vi "PH_4_Pos_Selector.ProcCases.vi"(0 "i ref in":refnum<vi>, 1 "selector":string, 2 "data":i8[](array[numeric]), 3 "call cluster":T1={"Object"="", "Selector"="", "CallType"=enum."synchronous", "Async Object"="", "Async Selector"="", "Data Descriptor"="", "Data"=[], "Error #"=0, "Expire"=0}, 5 "error in":errorcluster) -> (14 "i ref out":refnum<vi>, 17 "answer cluster":T1={"Object"="", "Selector"="", "CallType"=enum."synchronous", "Async Object"="", "Async Selector"="", "Data Descriptor"="", "Data"=[], "Error #"=0, "Expire"=0}, 19 "error out":errorcluster)   [LabVIEW 2014, in "PH_4_Pos_Selector.lvlib"]
doc: "This method is called by a process from within the default case in the event loop. The methods of a class that are linked to events will be called from THIS method. Add your code here."
uses:
  PH_4_Pos_Selector.lvlib
  CSCore/CSSystem/CoreDefs/CoreDefs.call_type.ctl
  CSCore/BaseProcess/BaseProcess.descriptor string definition.ctl
  CSCore/CSSystem/CoreDefs/CoreDefs.rawDataType.ctl
  PH_4_Pos_Selector.Position Selector.ctl
  CSCore/CSSystem/CoreLib/CoreLib.string 2 byte array.vi
  CSCore/CSSystem/CoreLib/CoreLib.byte array 2 short.vi
  PH_AxisGUI_6P/PH_AxisGUI_6P.lvlib
  CSCore/CSSystem/CoreLib/CoreLib.lvlib
  CSCore/BaseProcess/BaseProcess.lvlib
  CSCore/CAEObj/CAEObj.lvlib
  PH_PSDBWriter/PH_PSDBWriter.lvlib
  PH_Common/PH_Common.lvlib
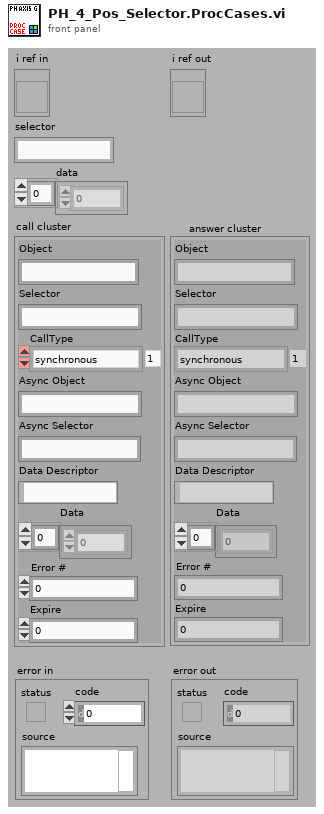
[diagram p1: front panel]
types:
  T1 = typedef "CoreDefs.call_type.ctl" = cluster{"Object":string, "Selector":string, "CallType":enum16{"simple", "synchronous", "asynchronous"}, "Async Object":string, "Async Selector":string, "Data Descriptor":T2, "Data":T3, "Error #":i32, "Expire":u32}
  T2 = typedef "BaseProcess.lvlib/BaseProcess.descriptor string definition.ctl" = string
  T3 = typedef "CoreDefs.rawDataType.ctl" = i8[]
  T4 = typedef "PH_PSDBWriter.lvlib/PH_PSDBWriter.PHELIX-Subsystems.ctl" = i32
  T5 = typedef "PH_4_Pos_Selector.lvlib/PH_4_Pos_Selector.Position Selector.ctl" = u16
  T6 = typedef "PH_4_Pos_Selector.lvlib/PH_4_Pos_Selector.i attribute.ctl" = cluster{"GUI Refs":cluster{"Position I":refnum<vi>, "Position II":refnum<vi>, "Position III":refnum<vi>, "Position IV":refnum<vi>, "rel. Mode?":refnum<vi>, "Define Selector":refnum<vi>}, "Current Position":T5, "Service ID Position":i32, "Position Array":T7[], "Description Array":string[], "relative Mode":bool, "Wanted Define Selector Position":string}
  T7 = typedef "PH_4_Pos_Selector.lvlib/PH_4_Pos_Selector.Position.ctl" = cluster{"Axis 1":dbl, "Axis 2":dbl}
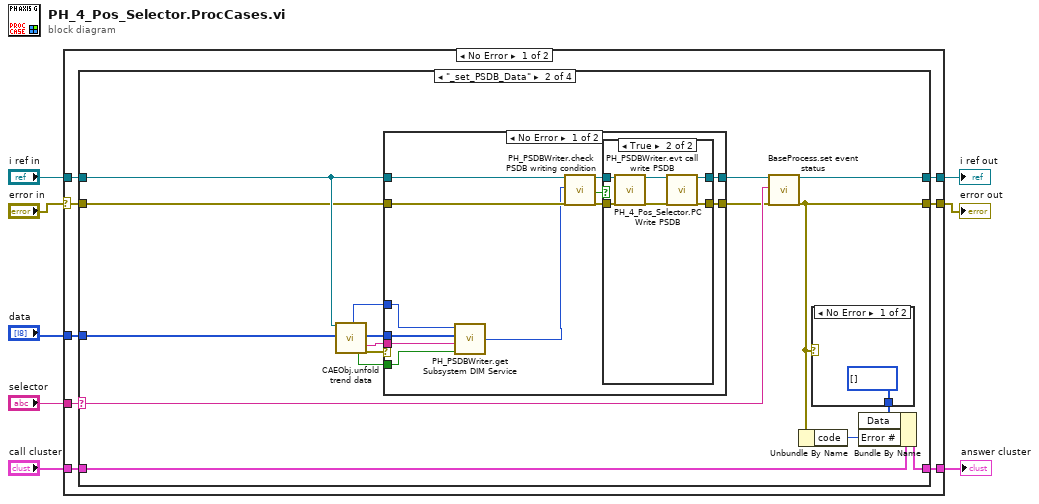
[diagram p0: block diagram]
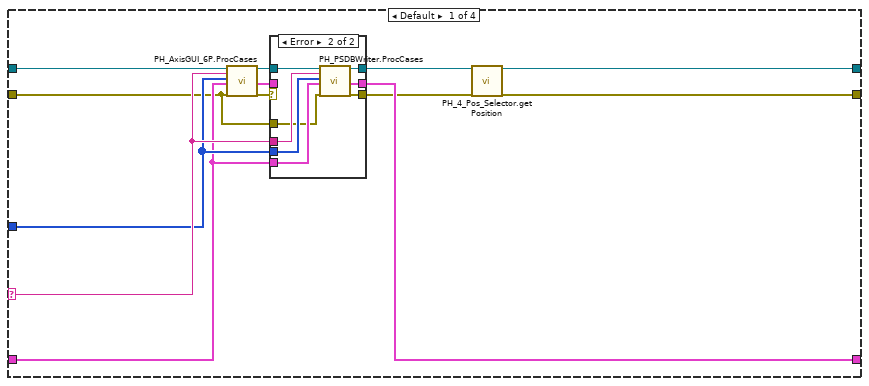
[diagram p2: hidden frame]
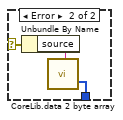
[diagram p6: hidden frame]
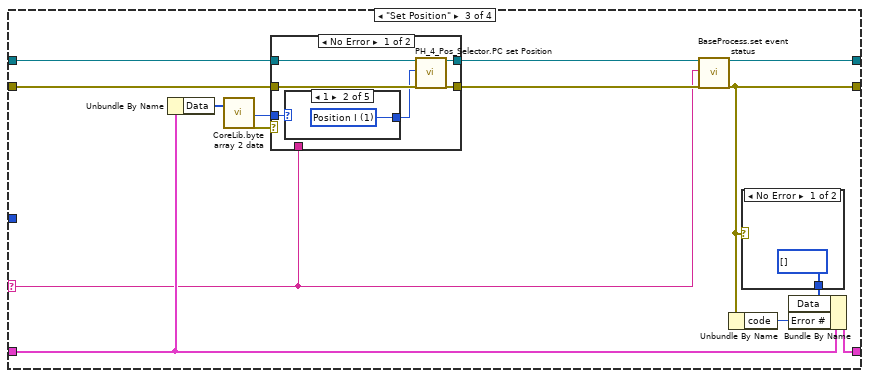
[diagram p7: hidden frame]
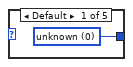
[diagram p8: hidden frame]
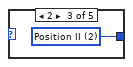
[diagram p9: hidden frame]
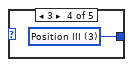
[diagram p10: hidden frame]
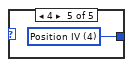
[diagram p11: hidden frame]
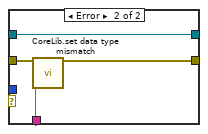
[diagram p12: hidden frame]
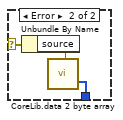
[diagram p13: hidden frame]
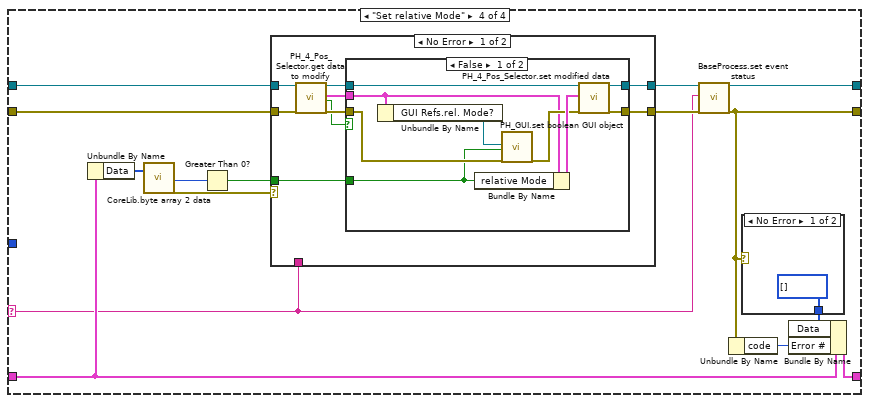
[diagram p14: hidden frame]
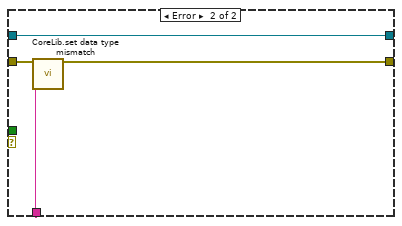
[diagram p16: hidden frame]
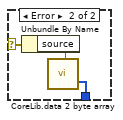
[diagram p17: hidden frame]
diagram:
  n1 = case shown="No Error" "error in" {
    selector: "error in" -> [w9 w161]
    tunnel: "selector" -> [w16 _]
    tunnel: [w15 w160] -> w7
    tunnel: "call cluster" -> [w14 w160]
    tunnel: "i ref in" -> [w13 w162]
    tunnel: [w12 w162] -> w4
    tunnel: [w11 w161] -> w3
    tunnel: "data" -> [w10 _]
    frame No Error {
      n2 = case shown="\"_set_PSDB_Data\"" w16 {
        selector: w16 -> [w26 w51 w85 w119]
        tunnel: w13 -> [w29 w45 w89 w123]
        tunnel: [w20 w55 w95 w129] -> w12
        tunnel: w14 -> [w24 w52 w91 w125]
        tunnel: [w23 w53 w93 w127] -> w15
        tunnel: w9 -> [w21 w41 w87 w121]
        tunnel: [w18 w54 w94 w128] -> w11
        tunnel: w10 -> [w25 w42 _ _]
        frame Default {
          n3 = call "PH_AxisGUI_6P.ProcCases.vi"("i ref in"=w29, "selector"=w26, "data"=w25, "call cluster"=w24, "error in"=w21) -> ("i ref out"=w28:refnum<vi>, "answer cluster"=w22:T1, "error out"=w27:errorcluster)  [unwired: 12 in]
          n4 = case shown="Error" w27 {
            selector: w27 -> [w31 _]
            tunnel: [w31 w40] -> w17
            tunnel: w28 -> [w32 w39]
            tunnel: [w32 w38] -> w19
            tunnel: w26 -> [_ w37]
            tunnel: w25 -> [_ w36]
            tunnel: w24 -> [_ w35]
            tunnel: [w30 w34] -> w23
            tunnel: w22 -> [w30 _]
            tunnel: w21 -> [_ w33]
            frame No Error {
            }
            frame Error {
              n5 = call "PH_PSDBWriter.ProcCases.vi"("i ref in"=w39, "selector"=w37, "Data"=w36, "call cluster"=w35, "error in"=w33) -> ("i ref out"=w38:refnum<vi>, "answer cluster"=w34:T1, "error out"=w40:errorcluster)  [unwired: 12 in]
            }
          }
          n6 = call "PH_4_Pos_Selector.get Position.vi"("i ref in"=w19, "error in (no error)"=w17) -> ("i ref out"=w20:refnum<vi>, "error out"=w18:errorcluster)  [unwired: 16 in]
        }
        frame "_set_PSDB_Data" {
          n7 = call "CAEObj.unfold trend data.vi"("i ref in"=w45, "raw trend data"=w42) -> ("quality"=w46:i32, "no link"=w49:bool, "data"=w47:i8[], "typeDescriptor"=w48:string, "error out"=w50:errorcluster)  [unwired: 9 in, 4 out]
          n8 = case shown="No Error" w50 {
            tunnel: w41 -> [w69 w79]
            tunnel: [w68 w78] -> w44
            tunnel: [w67 w79] -> w43
            tunnel: w45 -> [w65 w78]
            tunnel: w49 -> [w59 _]
            tunnel: w48 -> [w61 _]
            tunnel: w47 -> [w62 _]
            tunnel: w46 -> [w60 _]
            frame No Error {
              n9 = call "PH_PSDBWriter.get Subsystem DIM Service.vi"("no link"=w59, "typeDescriptor"=w61, "data"=w62, "quality"=w60) -> ("PHELIX Subsystems"=w58:T4)
              n10 = call "PH_PSDBWriter.check PSDB writing condition.vi"("i ref in"=w65, "wanted Subsystem"=w58, "error IO"=w69) -> ("i ref out"=w64:refnum<vi>, "write PSDB?"=w63:bool, "error out"=w66:errorcluster)  [unwired: 14 in]
              n11 = case shown="True" w63 {
                tunnel: w66 -> [w70 w77]
                tunnel: [w71 w74] -> w68
                tunnel: [w70 w72] -> w67
                tunnel: w64 -> [w71 w76]
                frame False {
                }
                frame True {
                  n12 = call "PH_4_Pos_Selector.PC Write PSDB.vi"("i ref in"=w76, "error IO"=w77) -> ("i ref out"=w75:refnum<vi>, "error out"=w73:errorcluster)  [unwired: 16 in]
                  n13 = call "PH_PSDBWriter.evt call write PSDB.vi"("i ref in"=w75, "error in (no error)"=w73) -> ("i ref out"=w74:refnum<vi>, "error out"=w72:errorcluster)  [unwired: 16 in]
                }
              }
            }
            frame Error {
            }
          }
          n14 = call "BaseProcess.set event status.vi"("i ref in"=w44, "EventStatus"=w51, "error in (no error)"=w43) -> ("i ref out"=w55:refnum<vi>, "error out"=w54:errorcluster)  [unwired: 14 in, 1 out]
          n15 = Unbundle By Name(w54) -> ("code"=w57:i32)
          n16 = case shown="No Error" w54 {
            selector: w54 -> [_ w83]
            tunnel: [T3 [] ("byteArray out") w81] -> w56
            frame No Error {
            }
            frame Error {
              n17 = Unbundle By Name(w83) -> ("source"=w82:string)
              n18 = call-poly "CoreLib.data 2 byte array.vi"("string"=w82) -> ("byteArray out"=w81:T3)  [unwired: 18 in]
            }
          }
          n19 = Bundle By Name(cluster=w52, "Data"=w56, "Error #"=w57) -> (w53:T1)
        }
        frame "Set Position" {
          n20 = Unbundle By Name(w91) -> ("Data"=w92:T3)
          n21 = call-poly "CoreLib.byte array 2 data.vi"("byteArray"=w92) -> ("i16"=w84:i16, "error out"=w90:errorcluster)  [unwired: 16 in, 1 out]
          n22 = case shown="No Error" w90 {
            tunnel: [w101 w112] -> w88
            tunnel: w89 -> [w103 w112]
            tunnel: w87 -> [w102 w111]
            tunnel: [w100 w110] -> w86
            tunnel: w85 -> [_ w109]
            tunnel: w84 -> [w99 _]
            frame No Error {
              n23 = case shown="1" w99 {
                tunnel: [w104 w105 w106 w107 w108] -> w98
                frame Default {
                  w104 = T5 0 items=["unknown", "Position I", "Position II", "Position III", "Position IV"] ("Wanted Position")
                }
                frame 1 {
                  w105 = T5 1 items=["unknown", "Position I", "Position II", "Position III", "Position IV"] ("Wanted Position")
                }
                frame 2 {
                  w106 = T5 2 items=["unknown", "Position I", "Position II", "Position III", "Position IV"] ("Wanted Position")
                }
                frame 3 {
                  w107 = T5 3 items=["unknown", "Position I", "Position II", "Position III", "Position IV"] ("Wanted Position")
                }
                frame 4 {
                  w108 = T5 4 items=["unknown", "Position I", "Position II", "Position III", "Position IV"] ("Wanted Position")
                }
              }
              n24 = call "PH_4_Pos_Selector.PC set Position.vi"("i ref in"=w103, "Wanted Position"=w98, "error IO"=w102) -> ("i ref out"=w101:refnum<vi>, "error out"=w100:errorcluster)  [unwired: 15 in]
            }
            frame Error {
              n25 = call "CoreLib.set data type mismatch.vi"("error in (no error)"=w111, "error source"=w109) -> ("error out"=w110:errorcluster)  [unwired: 17 in]
            }
          }
          n26 = call "BaseProcess.set event status.vi"("i ref in"=w88, "EventStatus"=w85, "error in (no error)"=w86) -> ("i ref out"=w95:refnum<vi>, "error out"=w94:errorcluster)  [unwired: 14 in, 1 out]
          n27 = Unbundle By Name(w94) -> ("code"=w97:i32)
          n28 = case shown="No Error" w94 {
            selector: w94 -> [_ w116]
            tunnel: [T3 [] ("byteArray out") w114] -> w96
            frame No Error {
            }
            frame Error {
              n29 = Unbundle By Name(w116) -> ("source"=w115:string)
              n30 = call-poly "CoreLib.data 2 byte array.vi"("string"=w115) -> ("byteArray out"=w114:T3)  [unwired: 18 in]
            }
          }
          n31 = Bundle By Name(cluster=w91, "Data"=w96, "Error #"=w97) -> (w93:T1)
        }
        frame "Set relative Mode" {
          n32 = Unbundle By Name(w125) -> ("Data"=w126:T3)
          n33 = call-poly "CoreLib.byte array 2 data.vi"("byteArray"=w126) -> ("i16"=w118:i16, "error out"=w124:errorcluster)  [unwired: 16 in, 1 out]
          n34 = Greater Than 0?(x=w118) -> (x > 0?=w117:bool)
          n35 = case shown="No Error" w124 {
            tunnel: [w135 w155] -> w122
            tunnel: w123 -> [w140 w155]
            tunnel: w121 -> [w139 w154]
            tunnel: [w137 w153] -> w120
            tunnel: w119 -> [_ w152]
            tunnel: w117 -> [w132 _]
            frame No Error {
              n36 = call "PH_4_Pos_Selector.get data to modify.vi"("i ref in"=w140, "error in (no error)"=w139) -> ("i ref out"=w136:refnum<vi>, "i attribute"=w133:T6, "timed out"=w134:bool, "error out"=w138:errorcluster)  [unwired: 14 in]
              n37 = case shown="False" w134 {
                tunnel: w138 -> [w149 w150]
                tunnel: [w148 w150] -> w137
                tunnel: w136 -> [w147 w151]
                tunnel: [w146 w151] -> w135
                tunnel: w133 -> [w143 _]
                tunnel: w132 -> [w141 _]
                frame False {
                  n38 = Unbundle By Name(w143) -> ("GUI Refs.rel. Mode?"=w142:refnum<vi>)
                  n39 = Bundle By Name(cluster=w143, "relative Mode"=w141) -> (w145:T6)
                  n40 = call "PH_GUI.set boolean GUI object.vi"("Boolean Knob GUI Ref"=w142, "Value"=w141, "error in (no error)"=w149) -> ("error out"=w144:errorcluster)  [unwired: 16 in]
                  n41 = call "PH_4_Pos_Selector.set modified data.vi"("i ref in"=w147, "i attribute"=w145, "error in (no error)"=w144) -> ("i ref out"=w146:refnum<vi>, "error out"=w148:errorcluster)  [unwired: 15 in]
                }
                frame True {
                }
              }
            }
            frame Error {
              n42 = call "CoreLib.set data type mismatch.vi"("error in (no error)"=w154, "error source"=w152) -> ("error out"=w153:errorcluster)  [unwired: 17 in]
            }
          }
          n43 = call "BaseProcess.set event status.vi"("i ref in"=w122, "EventStatus"=w119, "error in (no error)"=w120) -> ("i ref out"=w129:refnum<vi>, "error out"=w128:errorcluster)  [unwired: 14 in, 1 out]
          n44 = Unbundle By Name(w128) -> ("code"=w131:i32)
          n45 = case shown="No Error" w128 {
            selector: w128 -> [_ w159]
            tunnel: [T3 [] ("byteArray out") w157] -> w130
            frame No Error {
            }
            frame Error {
              n46 = Unbundle By Name(w159) -> ("source"=w158:string)
              n47 = call-poly "CoreLib.data 2 byte array.vi"("string"=w158) -> ("byteArray out"=w157:T3)  [unwired: 18 in]
            }
          }
          n48 = Bundle By Name(cluster=w125, "Data"=w130, "Error #"=w131) -> (w127:T1)
        }
      }
    }
    frame Error {
    }
  }
  "answer cluster" <- w7
  "i ref out" <- w4
  "error out" <- w3
